vi "Array_Investigation Part 2.vi"() -> ()   [LabVIEW 2014]
doc: "This VI is an exercise in the LabVIEW Core I course.\n\nEnter the number of columns and rows you want generated, then run the VI. This VI generates an array with the number of rows and columns you specify."
panel:
  out "Intensity Graph":dbl[][](graph)
  out "Array":dbl[][](array[numeric])
  in  "Rows":i32=80
  in  "Columns":i32=80
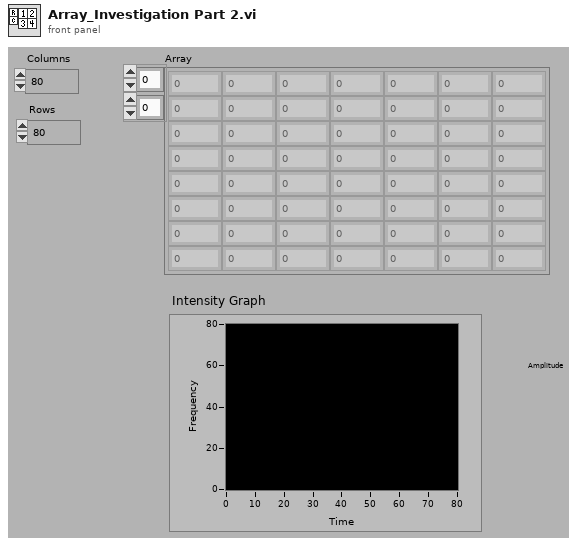
[diagram p1: front panel]
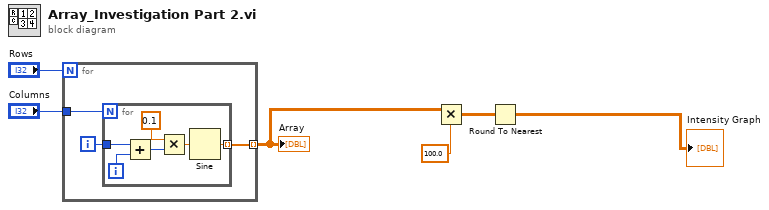
[diagram p0: block diagram]
diagram:
  n1 = for {
    N: "Rows" -> [_]
    tunnel: [w9] -> w4 mode=indexing
    tunnel: "Columns" -> [w8]
    i -> [w7]
    n2 = for {
      N: w8 -> [_]
      tunnel: [w15] -> w9 mode=indexing
      tunnel: w7 -> [w12]
      i -> [w13]
      n3 = Add(x=w12, y=w13) -> (x+y=w14:i32)
      n4 = Multiply(x=0.1, y=w14) -> (x*y=w11:dbl)
      n5 = Sine(x=w11) -> (sin(x)=w15:dbl)
    }
  }
  "Array" <- w4
  n6 = Multiply(x=w4, y=100.0) -> (x*y=w2:dbl[][])
  n7 = Round To Nearest(number=w2) -> (nearest integer value=→"Intensity Graph":dbl[][])
